vi "Test TDMS DAQmx.vi"() -> ()   [LabVIEW 2016]
uses:
  <vilib>/DAQmx/read.llb/DAQmx Read (Analog 1D Wfm NChan NSamp).vi
  <vilib>/DAQmx/create/channels.llb/DAQmx Create Channel (AI-Voltage-Basic).vi
  <vilib>/DAQmx/configure/task.llb/DAQmx Configure Logging (TDMS).vi
  <vilib>/DAQmx/configure/timing.llb/DAQmx Timing (Sample Clock).vi
  <vilib>/DAQmx/configure/trigger.llb/DAQmx Start Trigger (None).vi
  <vilib>/DAQmx/miscellaneous.llb/DAQmx Fill In Error Info.vi
panel:
  out "Waveform Graph 2":waveform(dbl)[](graph)
  in  "samples per channel":i32=1000
  in  "sample mode":i32(ring)=10178 items=["Finite Samples"=10178, "Continuous Samples"=10123, "Hardware Timed Single Point"=12522]
  in  "source":tag
  in  "rate":dbl=1000.0 format="%0.2f"
  in  "operation":i32(ring)=15846 items=["Open"=10437, "Open or Create"=15846, "Create or Replace"=15847, "Create"=15848]
  in  "logging mode":i32(ring)=15842 items=["Off"=10231, "Log"=15844, "Log and Read"=15842]
  in  "physical channels":tag
  out "names":string[](array[string])
  out "values":variant[](array[variant])
  out "Waveform Graph":waveform(dbl)(graph)
  in  "File Path Control":path=path "C:/Data/test.tdms"
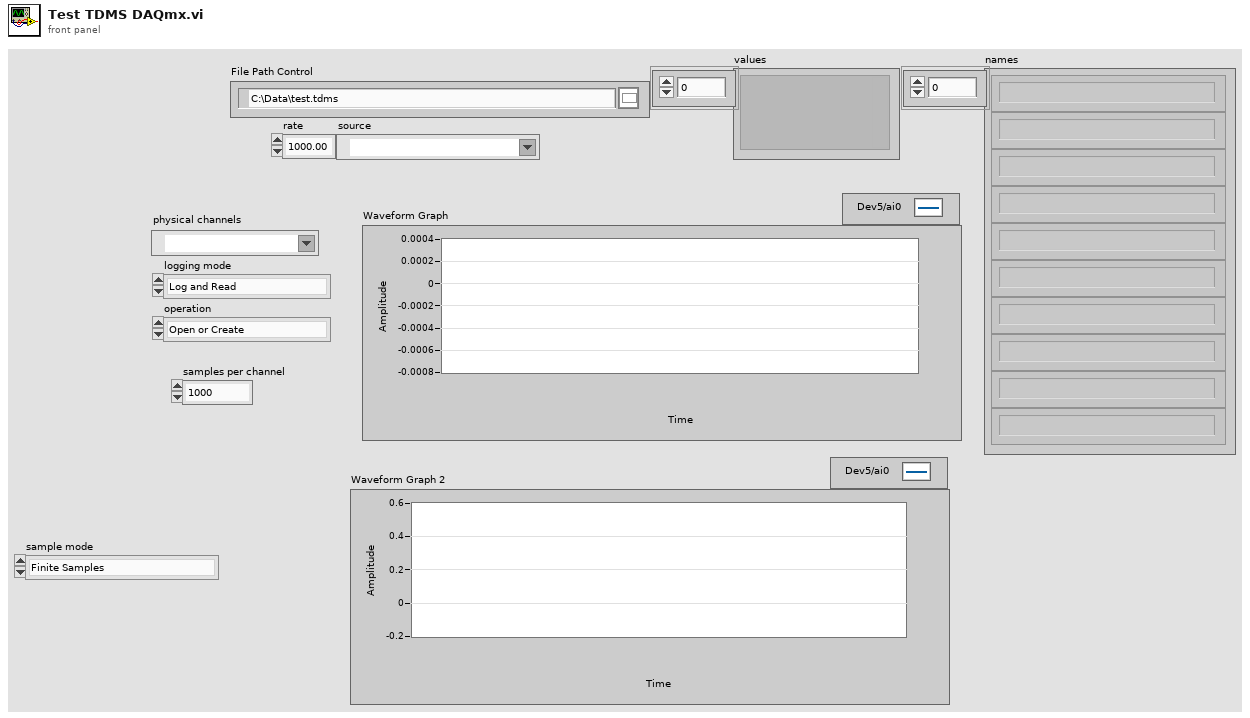
[diagram p1: front panel]
types:
  T1 = enum16{"open", "open or create", "create or replace", "create", "open (read-only)"}
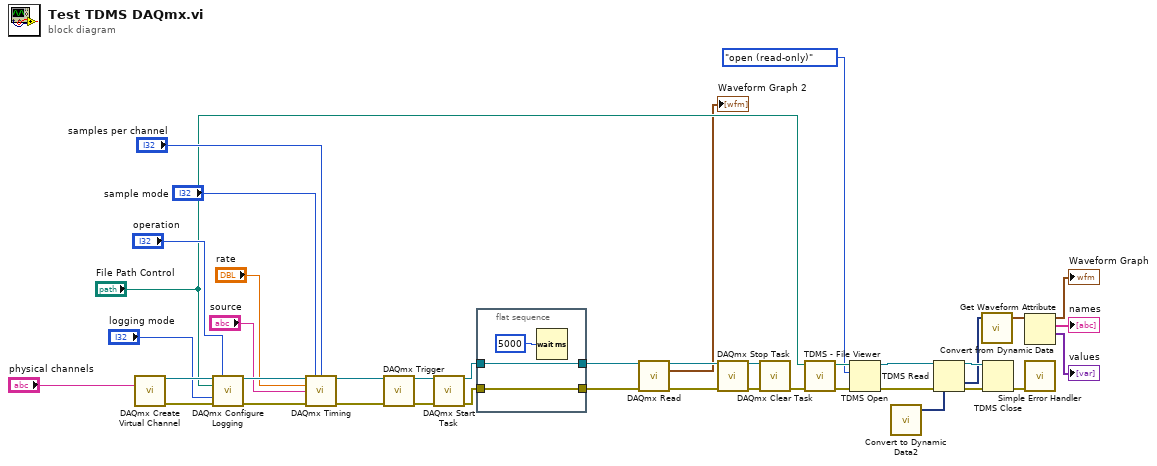
[diagram p0: block diagram]
diagram:
  n1 = call-poly <vilib>:"DAQmx Create Virtual Channel.vi"("physical channels"="physical channels") -> ("task out"=w25:refnum<k21>, "error out"=w22:errorcluster)  [unwired: 13 in]
  n2 = call-poly <vilib>:"DAQmx Configure Logging.vi"("task/channels in"=w25, "operation"="operation", "file path"="File Path Control", "logging mode"="logging mode", "error in"=w22) -> ("task out"=w21:refnum<k21>, "error out"=w20:errorcluster)  [unwired: 9 in]
  n3 = call-poly <vilib>:"DAQmx Timing.vi"("task/channels in"=w21, "sample mode"="sample mode", "samples per channel"="samples per channel", "rate"="rate", "source"="source", "error in"=w20) -> ("task out"=w14:refnum<k21>, "error out"=w15:errorcluster)  [unwired: 8 in]
  n4 = call-poly <vilib>:"DAQmx Trigger.vi"("task/channels in"=w14, "error in"=w15) -> ("task out"=w13:refnum<k21>, "error out"=w12:errorcluster)  [unwired: 12 in]
  n5 = call <vilib>:"DAQmx Start Task.vi"("task/channels in"=w13, "error in"=w12) -> ("task out"=w10:refnum<k21>, "error out"=w11:errorcluster)  [unwired: 12 in]
  n6 = flat-sequence {
    tunnel: w11 -> [w42]
    tunnel: w10 -> [w41]
    tunnel: [w42] -> w2
    tunnel: [w41] -> w9
    frame #0 {
      n7 = Wait (ms)(milliseconds to wait=u32 5000) -> ()  [unwired: 1 out]
    }
  }
  n8 = call-poly <vilib>:"DAQmx Read.vi"("task/channels in"=w9, "error in"=w2) -> ("task out"=w4:refnum<k21>, "data"=→"Waveform Graph 2":waveform(dbl)[], "error out"=w3:errorcluster)  [unwired: 11 in]
  n9 = call <vilib>:"DAQmx Stop Task.vi"("task/channels in"=w4, "error in"=w3) -> ("task out"=w8:refnum<k21>, "error out"=w7:errorcluster)  [unwired: 12 in]
  n10 = call <vilib>:"DAQmx Clear Task.vi"("task in"=w8, "error in"=w7) -> ("error out"=w6:errorcluster)  [unwired: 13 in]
  n11 = call <vilib>:"TDMS - File Viewer.vi"("error in (no error)"=w6, "file path"="File Path Control") -> ("error out"=w40:errorcluster, "file path out"=w39:path)  [unwired: 4 in]
  n12 = TDMS Open(8:w40, 10:T1."open (read-only)" ("operation (0:open)"), 11:w39) -> (0:w37:errorcluster, 3:w34:refnum<k34>)  [unwired: 4 in]
  n13 = call "Convert to Dynamic Data2"() -> ("Dynamic Data Type"=w32:dynamicdata)  [unwired: 4 in]
  n14 = TDMS Read(0:w34, 11:w37, 12:w32) -> (4:w33:refnum<k34>, 10:w31:dynamicdata, 15:w35:errorcluster)  [unwired: 5 in, 3 out]
  n15 = call "Convert from Dynamic Data"("Dynamic Data Type"=w31) -> ("Waveform"=w27:waveform(dbl))  [unwired: 3 in]
  n16 = TDMS Close(8:w35, 11:w33) -> (0:w36:errorcluster)  [unwired: 1 out]
  n17 = Get Waveform Attribute(7:w27) -> (1:→"values":variant[], 2:→"names":string[], 3:→"Waveform Graph":waveform(dbl))  [unwired: 3 in, 1 out]
  n18 = call <vilib>:"Simple Error Handler.vi"("error in (no error)"=w36) -> ()  [unwired: 4 in, 5 out]
